vi "lens_control_centrex_open_collector.vi"() -> ()   [LabVIEW 2017]
uses:
  <vilib>/Analysis/baseanly.llb/Mean (DBL).vi
  <vilib>/Utility/file.llb/Write Delimited Spreadsheet (string).vi
  <vilib>/Utility/file.llb/Write Delimited Spreadsheet (DBL).vi
  <vilib>/Analysis/NI_AALBase.lvlib
panel:
  out "size(s)":i32[](array[numeric])
  out "Voltage divider 2 (V)":dbl
  out "Voltage divider 1 (V)":dbl
  in  "Active":bool
  out "Initial time":dbl
  in  "Save data path":path=path "C:/Documents and Settings/EDM/Desktop/all_cond_argon_20kV_1x10-4.txt"
  in  "Save data?":bool=TRUE caption="Enable"
  out "Supply 2 Current":dbl(graph)
  out "Supply 1 Current":dbl(graph)
  out "Supply 2 Voltage":dbl(graph)
  out "Waveform Chart":dbl(graph)
  out "Loop iteration time":dbl
  in  "PS2 Set Voltage (kV)":dbl min=0.0 max=30.01 step=0.1 format="%.3f"
  in  "Both power supplies at\nsame voltage? (If true, \nPS1 voltage controls both supplies)":bool
  in  "Ramp time (s)":dbl
  out "relative seconds":dbl format="%_19f"
  out "time string":string
  out "date string":string
  out "Error Message":string="No Error"
  in  "Polarity switch 2 (ON = pos)":bool
  in  "Polarity switch 1 (ON = pos)":bool
  in  "POWER":bool
  in  "Stop":bool
  out "PS2 Voltage (kV)":dbl
  out "PS1 Voltage (kV)":dbl
  in  "PS1 Set Voltage (kV)":dbl min=0.0 max=30.01 step=0.1 format="%.3f"
  out "Ramp Step Size (kV)":dbl=0.025
  in  "Ramp Threshold (kV)":dbl=0.025
  in  "Ramp Voltage?":bool
  out "Supply 1 Voltage":dbl(graph)
  out "DeviceScanBacklog":i32
  out "LJMScanBacklog":i32=10
  out "Run Time":string="0  00:02:11" caption="Elapsed Time Text"
  out "Number of\nChannels":i32
  out "ScansPerRead":i32
  in  "Channels to Scan":string[](array[string])=["AIN0", "AIN1", "AIN2", "AIN3", "AIN4", "AIN5", "AIN6", "AIN7", "AIN8", "AIN9", "AIN10", "AIN11", "AIN12", "AIN13"]
  in  "Scan Rate (Hz)":dbl=150.0
  in  "Device type":string(combo)="Ethernet"
  in  "Connection Type":string(combo)="Ethernet"
  out "Connection Error on Start?":bool
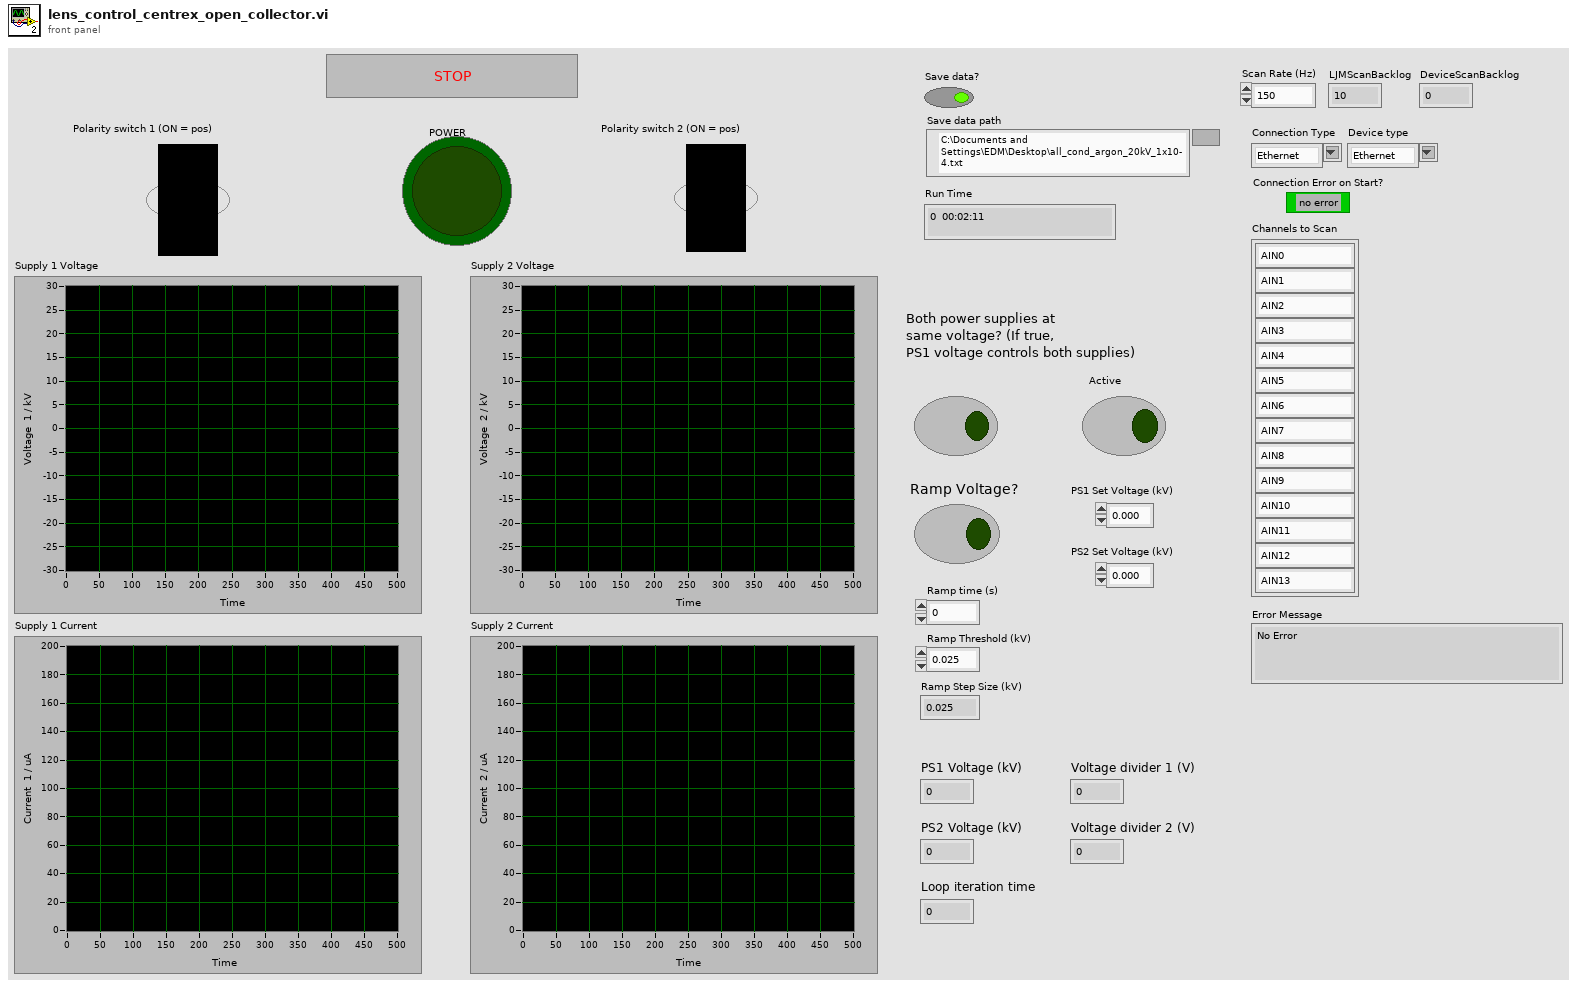
[diagram p1: front panel]
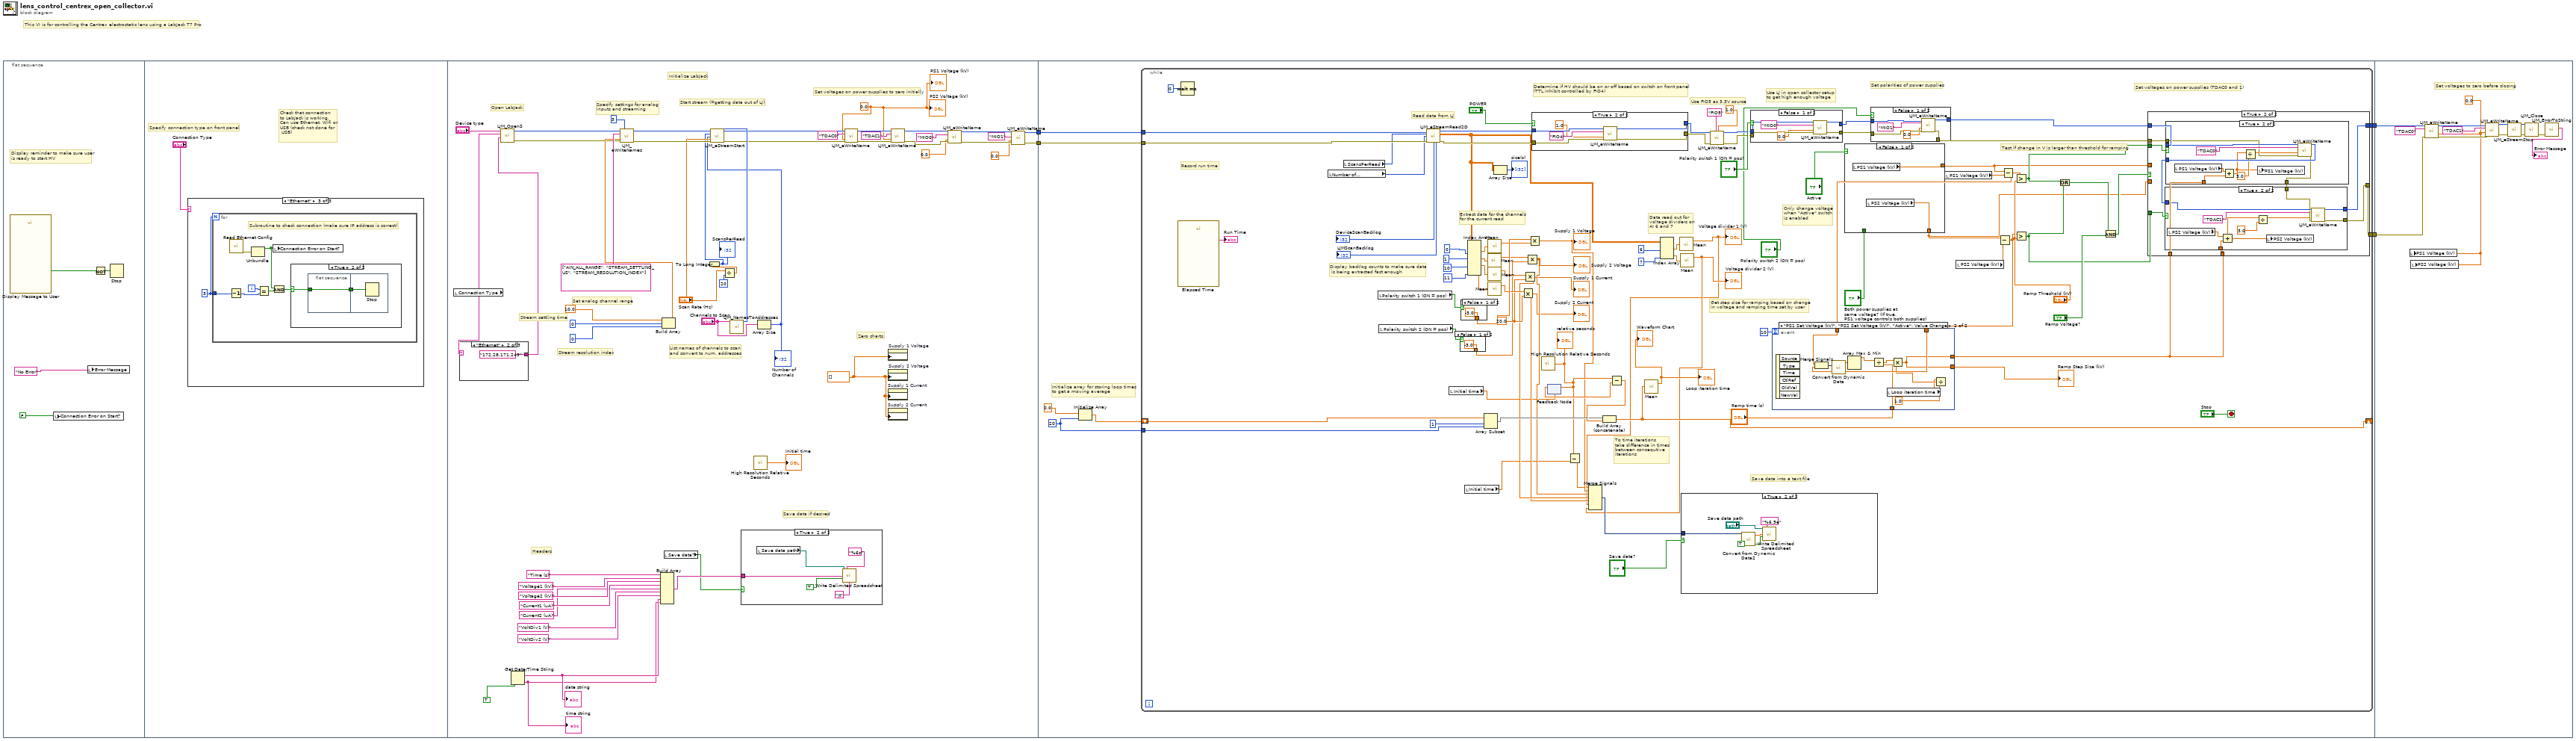
[diagram p0: block diagram]
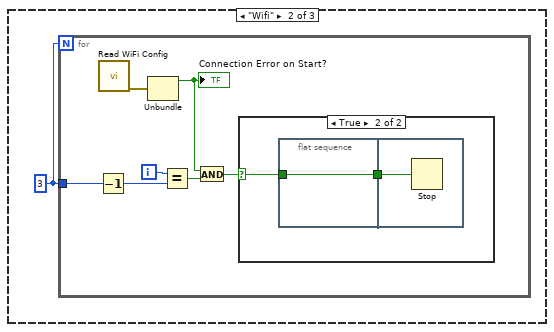
[diagram p3: hidden frame]
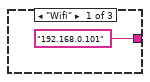
[diagram p7: hidden frame]
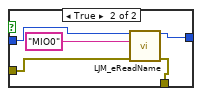
[diagram p9: hidden frame]
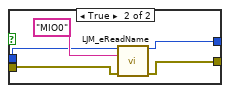
[diagram p10: hidden frame]
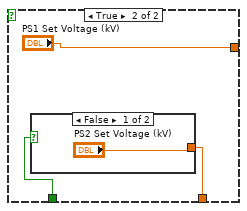
[diagram p11: hidden frame]
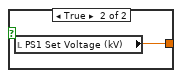
[diagram p12: hidden frame]
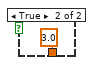
[diagram p13: hidden frame]
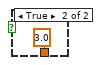
[diagram p14: hidden frame]
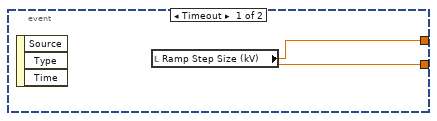
[diagram p16: hidden frame]
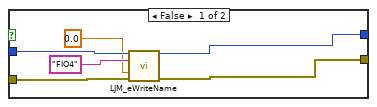
[diagram p17: hidden frame]
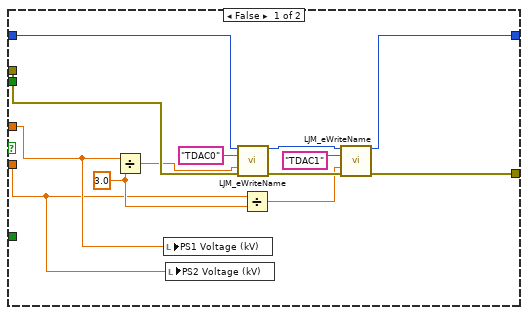
[diagram p18: hidden frame]
diagram:
  # "This VI is for controlling the Centrex electrostatic lens using a LabJack T7 Pro"
  n1 = flat-sequence {
    tunnel: [w50] -> w4
    tunnel: [w49] -> w3
    tunnel: w4 -> [w98]
    tunnel: w3 -> [w97]
    tunnel: [w96] -> w2
    tunnel: [w95] -> w1
    tunnel: w2 -> [w307]
    tunnel: w1 -> [w306]
    frame #0 {
      # "Display reminder to make sure user\nis ready to start HV"
      n2 = call "Display Message to User"() -> ("GO GO GO!"=w7:bool)  [unwired: 10 in, 1 out]
      n3 = local write "Connection Error on Start?"(FALSE) -> ()
      n4 = local write "Error Message"("No Error" ("Error Message")) -> ()
      n5 = Not(x=w7) -> (.not. x?=w8:bool)
      n6 = Stop(stop? (T)=w8) -> ()
    }
    frame #1 {
      # "Specify connection type on front panel"
      # "Check that connection\nto LabJack is working.\nCan use Ethernet, Wifi or\nUSB (check not done for\n USB)"
      n7 = case shown="\"Ethernet\"" "Connection Type" {
        frame Default {
        }
        frame "Wifi" {
          w10 = 3
          n8 = for {
            N: w10 -> [_]
            tunnel: w10 -> [w12]
            i -> [w14]
            n9 = Decrement(x=w12) -> (x-1=w11:i32)
            n10 = call "Read WiFi Config.vi"() -> ("error out"=w17:errorcluster)  [unwired: 11 in]
            n11 = Unbundle(w17) -> ("status"=w16:bool)  [unwired: 2 out]
            "Connection Error on Start?" <- w16
            n12 = Equal?(x=w14, y=w11) -> (x = y?=w15:bool)
            n13 = And(x=w16, y=w15) -> (x .and. y?=w13:bool)
            n14 = case shown="True" w13 {
              selector: w13 -> [_ w19]
              frame False {
              }
              frame True {
                n15 = flat-sequence {
                  tunnel: w19 -> [w20]
                  tunnel: [w20] -> w18
                  tunnel: w18 -> [w21]
                  frame #0 {
                  }
                  frame #1 {
                    n16 = Stop(stop? (T)=w21) -> ()
                  }
                }
              }
            }
          }
        }
        frame "Ethernet" {
          w22 = 3
          n17 = for {
            N: w22 -> [_]
            tunnel: w22 -> [w26]
            i -> [w28]
            # "Subroutine to check connection (make sure IP address is correct)"
            n18 = Decrement(x=w26) -> (x-1=w25:i32)
            n19 = call "Read Ethernet Config.vi"() -> ("error out"=w24:errorcluster)  [unwired: 11 in]
            n20 = Unbundle(w24) -> ("status"=w23:bool)  [unwired: 2 out]
            n21 = Equal?(x=w28, y=w25) -> (x = y?=w29:bool)
            n22 = And(x=w23, y=w29) -> (x .and. y?=w27:bool)
            n23 = local write "Connection Error on Start?"(w23) -> ()
            n24 = case shown="True" w27 {
              selector: w27 -> [_ w31]
              frame False {
              }
              frame True {
                n25 = flat-sequence {
                  tunnel: w31 -> [w32]
                  tunnel: [w32] -> w30
                  tunnel: w30 -> [w33]
                  frame #0 {
                  }
                  frame #1 {
                    n26 = Stop(stop? (T)=w33) -> ()
                  }
                }
              }
            }
          }
        }
      }
    }
    frame #2 {
      w39 = dbl[] [] ("History Data")
      w48 = 0.0
      # "Save data if desired"
      # "Headers"
      # "Stream resolution index"
      # "Stream settling time"
      # "Set analog channel range"
      # "Zero charts"
      # "Set voltages on power supplies to zero initially"
      # "List names of channels to scan\nand convert to num. addresses"
      # "Start stream (=getting data out of LJ)"
      # "Specify settings for analog \ninputs and streaming"
      # "Open LabJack"
      # "Initialize LabJack"
      n27 = local read "Connection Type"() -> (w83:string)
      n28 = case shown="\"Ethernet\"" w83 {
        tunnel: ["192.168.0.101" "172.28.171.249" _] -> w84
        frame "Wifi" {
        }
        frame "Ethernet" {
        }
        frame Default {
        }
      }
      n29 = call <userlib>:"LJM_OpenS.vi"("Identifier"=w84, "ConnectionType"=w83, "DeviceType"="Device type") -> ("error out"=w75:errorcluster, "Handle"=w76:i32)  [unwired: 7 in]
      n30 = Get Date/Time String(want seconds? (F)=TRUE) -> (date string=w35:string, time string=w34:string)  [unwired: 2 in]
      "date string" <- w35
      "time string" <- w34
      n31 = Build Array("Time (s)", "Voltage1 (kV)", "Voltage2 (kV)", "Current1 (uA)", "Current2 (uA)", "VoltDiv1 (V)", "VoltDiv2 (V)", w35, w34) -> (w42:string[])
      n32 = Build Array(10.0 ("Analog In Range (V)"), 0 ("Stream Settling Time (us)"), 0 ("Stream Resolution Index")) -> (w77:dbl[])
      n33 = call "LJM_eWriteNames.vi"("Handle In"=w76, "NumFrames"=3, "aNames"=string[] ["AIN_ALL_RANGE", "STREAM_SETTLING_US", "STREAM_RESOLUTION_INDEX"], "aValuesIn"=w77, "error in"=w75) -> ("Handle Out"=w67:i32, "error out"=w72:errorcluster)  [unwired: 8 in, 1 out]
      n34 = local read "Save data?"() -> (w41:bool)
      n35 = Divide(x="Scan Rate (Hz)", y=20) -> (x/y=w69:dbl)
      n36 = To Long Integer(number=w69) -> (32bit integer=w68:i32)
      "ScansPerRead" <- w68
      n37 = call <userlib>:"LJM_NamesToAddresses.vi"("aNames"="Channels to Scan") -> ("aAddresses"=w73:i32[])  [unwired: 8 in, 2 out]
      n38 = case shown="True" w41 {
        tunnel: w42 -> [_ w87]
        frame False {
        }
        frame True {
          n39 = local read "Save data path"() -> (w89:path)
          n40 = call-poly <vilib>:"Write Delimited Spreadsheet.vi"("file path (dialog if empty)"=w89, "format (%s)"="%6s" ("format (%.3f)"), "1D data"=w87, "append to file? (new file:F)"=TRUE, "delimiter (\\t)"="\t") -> ()  [unwired: 9 in, 2 out]
        }
      }
      n41 = call <vilib>:"High Resolution Relative Seconds.vi"() -> ("relative seconds"=→"Initial time":dbl)
      n42 = Array Size(array="Channels to Scan") -> (size(s)=w65:i32)
      "Number of\nChannels" <- w65
      n43 = call "LJM_eStreamStart.vi"("Handle In"=w67, "aScanList"=w73, "ScansPerRead"=w68, "NumAddresses"=w65, "ScanRate"="Scan Rate (Hz)", "error in"=w72) -> ("Handle Out"=w64:i32, "error out"=w63:errorcluster)  [unwired: 7 in, 1 out]
      n44 = call <userlib>:"LJM_eWriteName.vi"("Handle In"=w64, "Name"="TDAC0", "Value"=w48, "error in"=w63) -> ("Handle Out"=w60:i32, "error out"=w61:errorcluster)  [unwired: 10 in]
      n45 = property on="Supply 1 Current" class="WFChart (strict)"("History Data"=w39) -> ()  [unwired: 2 in, 2 out]
      n46 = property on="Supply 2 Current" class="WFChart (strict)"("History Data"=w39) -> ()  [unwired: 2 in, 2 out]
      n47 = property on="Supply 1 Voltage" class="WFChart (strict)"("History Data"=w39) -> ()  [unwired: 2 in, 2 out]
      n48 = property on="Supply 2 Voltage" class="WFChart (strict)"("History Data"=w39) -> ()  [unwired: 2 in, 2 out]
      n49 = call <userlib>:"LJM_eWriteName.vi"("Handle In"=w60, "Name"="TDAC1", "Value"=w48, "error in"=w61) -> ("Handle Out"=w57:i32, "error out"=w58:errorcluster)  [unwired: 10 in]
      n50 = call <userlib>:"LJM_eWriteName.vi"("Handle In"=w57, "Name"="MIO0", "Value"=0.0, "error in"=w58) -> ("Handle Out"=w56:i32, "error out"=w53:errorcluster)  [unwired: 10 in]
      n51 = call <userlib>:"LJM_eWriteName.vi"("Handle In"=w56, "Name"="MIO1", "Value"=0.0, "error in"=w53) -> ("Handle Out"=w50:i32, "error out"=w49:errorcluster)  [unwired: 10 in]
      "PS1 Voltage (kV)" <- w48
      "PS2 Voltage (kV)" <- w48
    }
    frame #3 {
      w92 = 20
      # "Initialize array for storing loop times\nto get a moving average"
      n52 = Initialize Array(0.0, w92) -> (w93:dbl[])
      n53 = while {
        tunnel: w98 -> [w184]
        tunnel: w97 -> [w183]
        tunnel: [w166] -> w96
        tunnel: [w165] -> w95
        shift-right: [w156] -> _
        shift-left: w93 -> [w154]
        tunnel: w92 -> [w151]
        stop <- "Stop" stop-if-true
        w142 = 20.0
        # "Use LJ in open collector setup\nto get high enough voltage"
        # "Only change voltage\nwhen \"Active\" switch\nis enabled"
        # "Set polarities of power supplies"
        # "Use FIO5 as 3.3V source"
        # "To time iterations\ntake difference in times\nbetween consequtive\niterations"
        # "Save data into a text file"
        # "Data read out for \nvoltage dividers on\nAI 6 and 7"
        # "Get step size for ramping based on change\nin voltage and ramping time set by user"
        # "Determine if HV should be on or off based on switch on front panel\n(TTL inhibit controlled by FIO4)"
        # "Test if change in V is larger than threshold for ramping"
        # "Set voltages on power supplies (TDAC0 and 1)"
        # "Extract data for the channels\nfor the current read"
        # "Display backlog counts to make sure data\n is being extracted fast enough"
        # "Record run time"
        # "Read data from LJ"
        n54 = call "Elapsed Time"() -> ("Elapsed Time Text"=→"Run Time":string)  [unwired: 12 in, 7 out]
        n55 = Wait (ms)(milliseconds to wait=0) -> ()  [unwired: 1 out]
        n56 = local read "Number of\nChannels"() -> (w181:i32)
        n57 = local read "ScansPerRead"() -> (w182:i32)
        n58 = local read "Polarity switch 1 (ON = pos)"() -> (w130:bool)
        n59 = local read "Polarity switch 2 (ON = pos)"() -> (w129:bool)
        n60 = call "LJM_eStreamRead2D.vi"("Handle In"=w184, "ScansPerRead"=w182, "NumAddresses"=w181, "error in"=w183) -> ("Handle Out"=w168:i32, "aData Out"=w121:dbl[][], "DeviceScanBacklog"=→"DeviceScanBacklog":i32, "LJMScanBacklog"=→"LJMScanBacklog":i32, "error out"=w169:errorcluster)  [unwired: 7 in]
        n61 = local read "Initial time"() -> (w113:dbl)
        n62 = case shown="False" w129 {
          tunnel: [-3.0 3.0] -> w128
          frame False {
          }
          frame True {
          }
        }
        n63 = case shown="False" w130 {
          tunnel: [-3.0 3.0] -> w145
          frame False {
          }
          frame True {
          }
        }
        n64 = local read "Initial time"() -> (w131:dbl)
        n65 = Index Array(array=w121, index (col) #1=0, index (col) #2=1, index (col) #3=10, index (col) #4=11) -> (element #1=w164:dbl[], element #2=w150:dbl[], element #3=w149:dbl[], element #4=w148:dbl[])  [unwired: 4 in]
        n66 = Array Subset(array=w154, index=1, length=w151) -> (w153:dbl[])
        n67 = call-poly <vilib>:"Mean.vi"("X"=w150) -> ("mean"=w140:dbl)  [unwired: 1 out]
        n68 = call-poly <vilib>:"Mean.vi"("X"=w164) -> ("mean"=w141:dbl)  [unwired: 1 out]
        n69 = call-poly <vilib>:"Mean.vi"("X"=w149) -> ("mean"=w144:dbl)  [unwired: 1 out]
        n70 = call-poly <vilib>:"Mean.vi"("X"=w148) -> ("mean"=w143:dbl)  [unwired: 1 out]
        n71 = Array Size(array=w121) -> (size(s)=→"size(s)":i32[])
        n72 = Multiply(x=w143, y=w142) -> (x*y=w135:dbl)
        "Supply 2 Current" <- w135
        n73 = Multiply(x=w144, y=w142) -> (x*y=w136:dbl)
        "Supply 1 Current" <- w136
        n74 = Multiply(x=w140, y=w128) -> (x*y=w137:dbl)
        "Supply 2 Voltage" <- w137
        n75 = Multiply(x=w145, y=w141) -> (x*y=w138:dbl)
        "Supply 1 Voltage" <- w138
        n76 = case shown="True" "POWER" {
          tunnel: w168 -> [w240 w246]
          tunnel: [w236 w243] -> w110
          tunnel: w169 -> [w239 w245]
          tunnel: [w237 w242] -> w111
          frame False {
            n77 = call <userlib>:"LJM_eWriteName.vi"("Handle In"=w240, "Name"="FIO4", "Value"=0.0, "error in"=w239) -> ("Handle Out"=w237:i32, "error out"=w236:errorcluster)  [unwired: 10 in]
          }
          frame True {
            n78 = call <userlib>:"LJM_eWriteName.vi"("Handle In"=w246, "Name"="FIO4", "Value"=1.0, "error in"=w245) -> ("Handle Out"=w242:i32, "error out"=w243:errorcluster)  [unwired: 10 in]
          }
        }
        n79 = call <vilib>:"High Resolution Relative Seconds.vi"() -> ("relative seconds"=w139:dbl)
        "relative seconds" <- w139
        n80 = feedback-in #1(w139) -> ()
        n81 = feedback #1(w113) -> (w158:dbl)
        n82 = Subtract(x=w139, y=w131) -> (x-y=w132:dbl)
        n83 = Subtract(x=w139, y=w158) -> (x-y=w157:dbl)
        n84 = Build Array (concatenate)(w153, w157) -> (w156:dbl[])
        n85 = call-poly <vilib>:"Mean.vi"("X"=w156) -> ("mean"=→"Loop iteration time" →"Waveform Chart":dbl)  [unwired: 1 out]
        n86 = Index Array(array=w121, index (col) #1=6, index (col) #2=7) -> (element #1=w123:dbl[], element #2=w122:dbl[])  [unwired: 2 in]
        n87 = call-poly <vilib>:"Mean.vi"("X"=w123) -> ("mean"=w107:dbl)  [unwired: 1 out]
        "Voltage divider 1 (V)" <- w107
        n88 = call-poly <vilib>:"Mean.vi"("X"=w122) -> ("mean"=w108:dbl)  [unwired: 1 out]
        "Voltage divider 2 (V)" <- w108
        n89 = Merge Signals(w132, w138, w137, w136, w135, w107, w108) -> (w133:dynamicdata)
        n90 = case shown="True" "Save data?" {
          tunnel: w133 -> [_ w222]
          frame False {
          }
          frame True {
            n91 = call "Convert from Dynamic Data2"("Dynamic Data Type"=w222) -> ("Array"=w221:dbl[])  [unwired: 3 in]
            n92 = call-poly <vilib>:"Write Delimited Spreadsheet.vi"("file path (dialog if empty)"="Save data path", "format (%.3f)"="%6.5e", "1D data"=w221, "append to file? (new file:F)"=TRUE) -> ()  [unwired: 10 in, 2 out]
          }
        }
        n93 = call <userlib>:"LJM_eWriteName.vi"("Handle In"=w111, "Name"="FIO5", "Value"=1.0, "error in"=w110) -> ("Handle Out"=w105:i32, "error out"=w104:errorcluster)  [unwired: 10 in]
        n94 = case shown="False" "Polarity switch 1 (ON = pos)" {
          tunnel: w105 -> [w202 w206]
          tunnel: w104 -> [w201 w205]
          tunnel: [w200 w203] -> w102
          tunnel: [w199 w204] -> w101
          frame False {
            n95 = call <userlib>:"LJM_eWriteName.vi"("Handle In"=w202, "Name"="MIO0", "Value"=0.0, "error in"=w201) -> ("Handle Out"=w200:i32, "error out"=w199:errorcluster)  [unwired: 10 in]
          }
          frame True {
            n96 = call "LJM_eReadName.vi"("Handle In"=w206, "Name"="MIO0", "error in"=w205) -> ("Handle Out"=w203:i32, "error out"=w204:errorcluster)  [unwired: 10 in, 1 out]
          }
        }
        n97 = case shown="False" "Active" {
          tunnel: [w209 "PS1 Set Voltage (kV)"] -> w127
          tunnel: "Both power supplies at\nsame voltage? (If true, \nPS1 voltage controls both supplies)" -> [_ w211]
          tunnel: [w208 w210] -> w125
          frame False {
            n98 = local read "PS1 Voltage (kV)"() -> (w209:dbl)
            n99 = local read "PS2 Voltage (kV)"() -> (w208:dbl)
          }
          frame True {
            n100 = case shown="False" w211 {
              tunnel: ["PS2 Set Voltage (kV)" w214] -> w210
              frame False {
              }
              frame True {
                n101 = local read "PS1 Set Voltage (kV)"() -> (w214:dbl)
              }
            }
          }
        }
        n102 = case shown="False" "Polarity switch 2 (ON = pos)" {
          tunnel: w102 -> [w191 w195]
          tunnel: w101 -> [w189 w192]
          tunnel: [w188 w194] -> w100
          tunnel: [w187 w193] -> w99
          frame False {
            n103 = call <userlib>:"LJM_eWriteName.vi"("Handle In"=w191, "Name"="MIO1", "Value"=0.0, "error in"=w189) -> ("Handle Out"=w188:i32, "error out"=w187:errorcluster)  [unwired: 10 in]
          }
          frame True {
            n104 = call "LJM_eReadName.vi"("Handle In"=w195, "Name"="MIO0", "error in"=w192) -> ("Handle Out"=w194:i32, "error out"=w193:errorcluster)  [unwired: 10 in, 1 out]
          }
        }
        n105 = local read "PS1 Voltage (kV)"() -> (w175:dbl)
        n106 = local read "PS2 Voltage (kV)"() -> (w174:dbl)
        n107 = Subtract(x=w125, y=w174) -> (x-y=w162:dbl)
        n108 = Subtract(x=w127, y=w175) -> (x-y=w163:dbl)
        n109 = event shown="[1] \"PS1 Set Voltage (kV)\", \"PS2 Set Voltage (kV)\", \"Active\": Value Change" {
          selector: _ -> [_ _]
          dyn-events: _ -> [_ _]
          timeout: 10 -> [_ _]
          tunnel: w163 -> [_ w235]
          tunnel: w162 -> [_ w234]
          tunnel: "Ramp time (s)" -> [_ w230]
          tunnel: [w224 w228] -> w160
          tunnel: [w224 w228] -> w159
          event Timeout {
            n110 = event-data() -> ()  [unwired: 1 in, 3 out]
            n111 = local read "Ramp Step Size (kV)"() -> (w224:dbl)
          }
          event "PS1 Set Voltage (kV)", "PS2 Set Voltage (kV)", "Active": Value Change {
            n112 = event-data() -> ()  [unwired: 1 in, 6 out]
            n113 = Merge Signals(w235, w234) -> (w233:dynamicdata)
            n114 = call "Convert from Dynamic Data"("Dynamic Data Type"=w233) -> ("Array"=w232:dbl[])  [unwired: 3 in]
            n115 = Array Max & Min(array=w232) -> (max value=w231:dbl)  [unwired: 3 out]
            n116 = Divide(x=w231, y=w230) -> (x/y=w229:dbl)
            n117 = local read "Loop iteration time"() -> (w226:dbl)
            n118 = Divide(x=w226, y=1.0) -> (x/y=w227:dbl)
            n119 = Multiply(x=w229, y=w227) -> (x*y=w228:dbl)
          }
        }
        "Ramp Step Size (kV)" <- w160
        n120 = Greater?(x=w163, y="Ramp Threshold (kV)") -> (0:w172:bool)
        n121 = Greater?(x=w162, y="Ramp Threshold (kV)") -> (0:w171:bool)
        n122 = Or(x=w172, y=w171) -> (x .or. y?=w176:bool)
        n123 = And(x=w176, y="Ramp Voltage?") -> (x .and. y?=w177:bool)
        n124 = case shown="True" w177 {
          tunnel: w100 -> [w259 w268]
          tunnel: w99 -> [w255 w266]
          tunnel: w125 -> [w250 _]
          tunnel: w127 -> [w251 _]
          tunnel: w172 -> [_ w270]
          tunnel: w171 -> [_ w269]
          tunnel: w159 -> [_ w264]
          tunnel: w159 -> [_ w263]
          tunnel: [w249 w262] -> w166
          tunnel: [w248 w261] -> w165
          frame False {
            w252 = 3.0
            n125 = Divide(x=w251, y=w252) -> (x/y=w253:dbl)
            n126 = local write "PS1 Voltage (kV)"(w251) -> ()
            n127 = local write "PS2 Voltage (kV)"(w250) -> ()
            n128 = call <userlib>:"LJM_eWriteName.vi"("Handle In"=w259, "Name"="TDAC0", "Value"=w253, "error in"=w255) -> ("Handle Out"=w257:i32, "error out"=w256:errorcluster)  [unwired: 10 in]
            n129 = Divide(x=w250, y=w252) -> (x/y=w254:dbl)
            n130 = call <userlib>:"LJM_eWriteName.vi"("Handle In"=w257, "Name"="TDAC1", "Value"=w254, "error in"=w256) -> ("Handle Out"=w249:i32, "error out"=w248:errorcluster)  [unwired: 10 in]
          }
          frame True {
            n131 = case shown="True" w270 {
              tunnel: w268 -> [w284 w294]
              tunnel: [w284 w293] -> w267
              tunnel: w266 -> [w283 w291]
              tunnel: [w283 w290] -> w265
              tunnel: w264 -> [_ w289]
              frame False {
              }
              frame True {
                n132 = local read "PS1 Voltage (kV)"() -> (w288:dbl)
                n133 = Add(x=w288, y=w289) -> (x+y=w285:dbl)
                n134 = Divide(x=w285, y=3.0) -> (x/y=w287:dbl)
                n135 = local write "PS1 Voltage (kV)"(w285) -> ()
                n136 = call <userlib>:"LJM_eWriteName.vi"("Handle In"=w294, "Name"="TDAC0", "Value"=w287, "error in"=w291) -> ("Handle Out"=w293:i32, "error out"=w290:errorcluster)  [unwired: 10 in]
              }
            }
            n137 = case shown="True" w269 {
              tunnel: w267 -> [w272 w282]
              tunnel: w265 -> [w271 w281]
              tunnel: w263 -> [_ w278]
              tunnel: [w272 w277] -> w262
              tunnel: [w271 w276] -> w261
              frame False {
              }
              frame True {
                n138 = local read "PS2 Voltage (kV)"() -> (w279:dbl)
                n139 = Add(x=w279, y=w278) -> (x+y=w273:dbl)
                n140 = Divide(x=w273, y=3.0) -> (x/y=w275:dbl)
                n141 = local write "PS2 Voltage (kV)"(w273) -> ()
                n142 = call <userlib>:"LJM_eWriteName.vi"("Handle In"=w282, "Name"="TDAC1", "Value"=w275, "error in"=w281) -> ("Handle Out"=w277:i32, "error out"=w276:errorcluster)  [unwired: 10 in]
              }
            }
          }
        }
      }
    }
    frame #4 {
      w301 = 0.0 ("Value")
      # "Set voltages to zero before closing"
      n143 = local write "PS1 Voltage (kV)"(w301) -> ()
      n144 = local write "PS2 Voltage (kV)"(w301) -> ()
      n145 = call <userlib>:"LJM_eWriteName.vi"("Handle In"=w307, "Name"="TDAC0", "Value"=w301, "error in"=w306) -> ("Handle Out"=w304:i32, "error out"=w303:errorcluster)  [unwired: 10 in]
      n146 = call <userlib>:"LJM_eWriteName.vi"("Handle In"=w304, "Name"="TDAC1", "Value"=w301, "error in"=w303) -> ("Handle Out"=w300:i32, "error out"=w296:errorcluster)  [unwired: 10 in]
      n147 = call "LJM_eStreamStop.vi"("Handle In"=w300, "error in"=w296) -> ("Handle Out"=w299:i32, "error out"=w297:errorcluster)  [unwired: 12 in]
      n148 = call <userlib>:"LJM_Close.vi"("error in"=w297, "Handle"=w299) -> ("error out"=w298:errorcluster)  [unwired: 9 in]
      n149 = call <userlib>:"LJM_ErrorToString.vi"("error in"=w298) -> ("String"=→"Error Message":string)  [unwired: 10 in]
    }
  }
